vi "HXG2_AlldataToArray.vi"(8 "error in (no error)":errorcluster, 9 "Calculated Values":T1, 10 "Analog In":T2) -> (0 "error out":errorcluster, 2 "Strings Out":string[](array[string])=["Liq In Avg", "Liq In 1", "Liq In 2", "Liq Out Avg", "Liq Out 1", "Liq Out 2", "Fltrd Mdot", "Liq Mdot", "Liq T° f/mtr", "Liq dP 0-25psi", "Liq Pin 0-100psi", "Air In Avg", "Air In 1", "Air In 2", "Air In 3", "Air In 4", "Air Out Avg", "Air Out 1", "Air Out 2", "Air Out 3", "Air Out 4", "Air Out 5", "Air Out 6", "Air Out 7", "Air Out 8", "CFM Nozzle", "CFM HX", "UUT 0-0.1inWC x100", "Chmb 0-5inWC x100", "Chmb 0-2.5inWC x100", "Liq Q (BTU/hr)", "Liq Q (W)", "Air Q (BTU/hr)", "Air Q (W)", "SH (°F)", "SH multiplier", "%Energy Bal", "Liq Re", "AF Ctl Out", "AC Ctl Out", "AH Ctl Out", "LF Ctl Out", "LC Ctl Out", "LH Ctl Out", "Box Btm In (9)", "Box Btm Out (10)", "Box Rt In (11)", "Box Rt Frt (12) ", "Box Top In(13)", "Box Top Out(14)", "Box Lt In (15)", "Box Lt Out (16)"], 3 "Plot":dbl[](array[numeric]))   [LabVIEW 2012]
uses:
  Controls/HXG2_AnalogIn.ctl
  Controls/HXG2_Calculated.ctl
  Modules/PID/HXG2pid.ctl
panel:
  out "element":string
  in  "index":i32=43
  out "Text Array":i32
  out "Number Array":i32
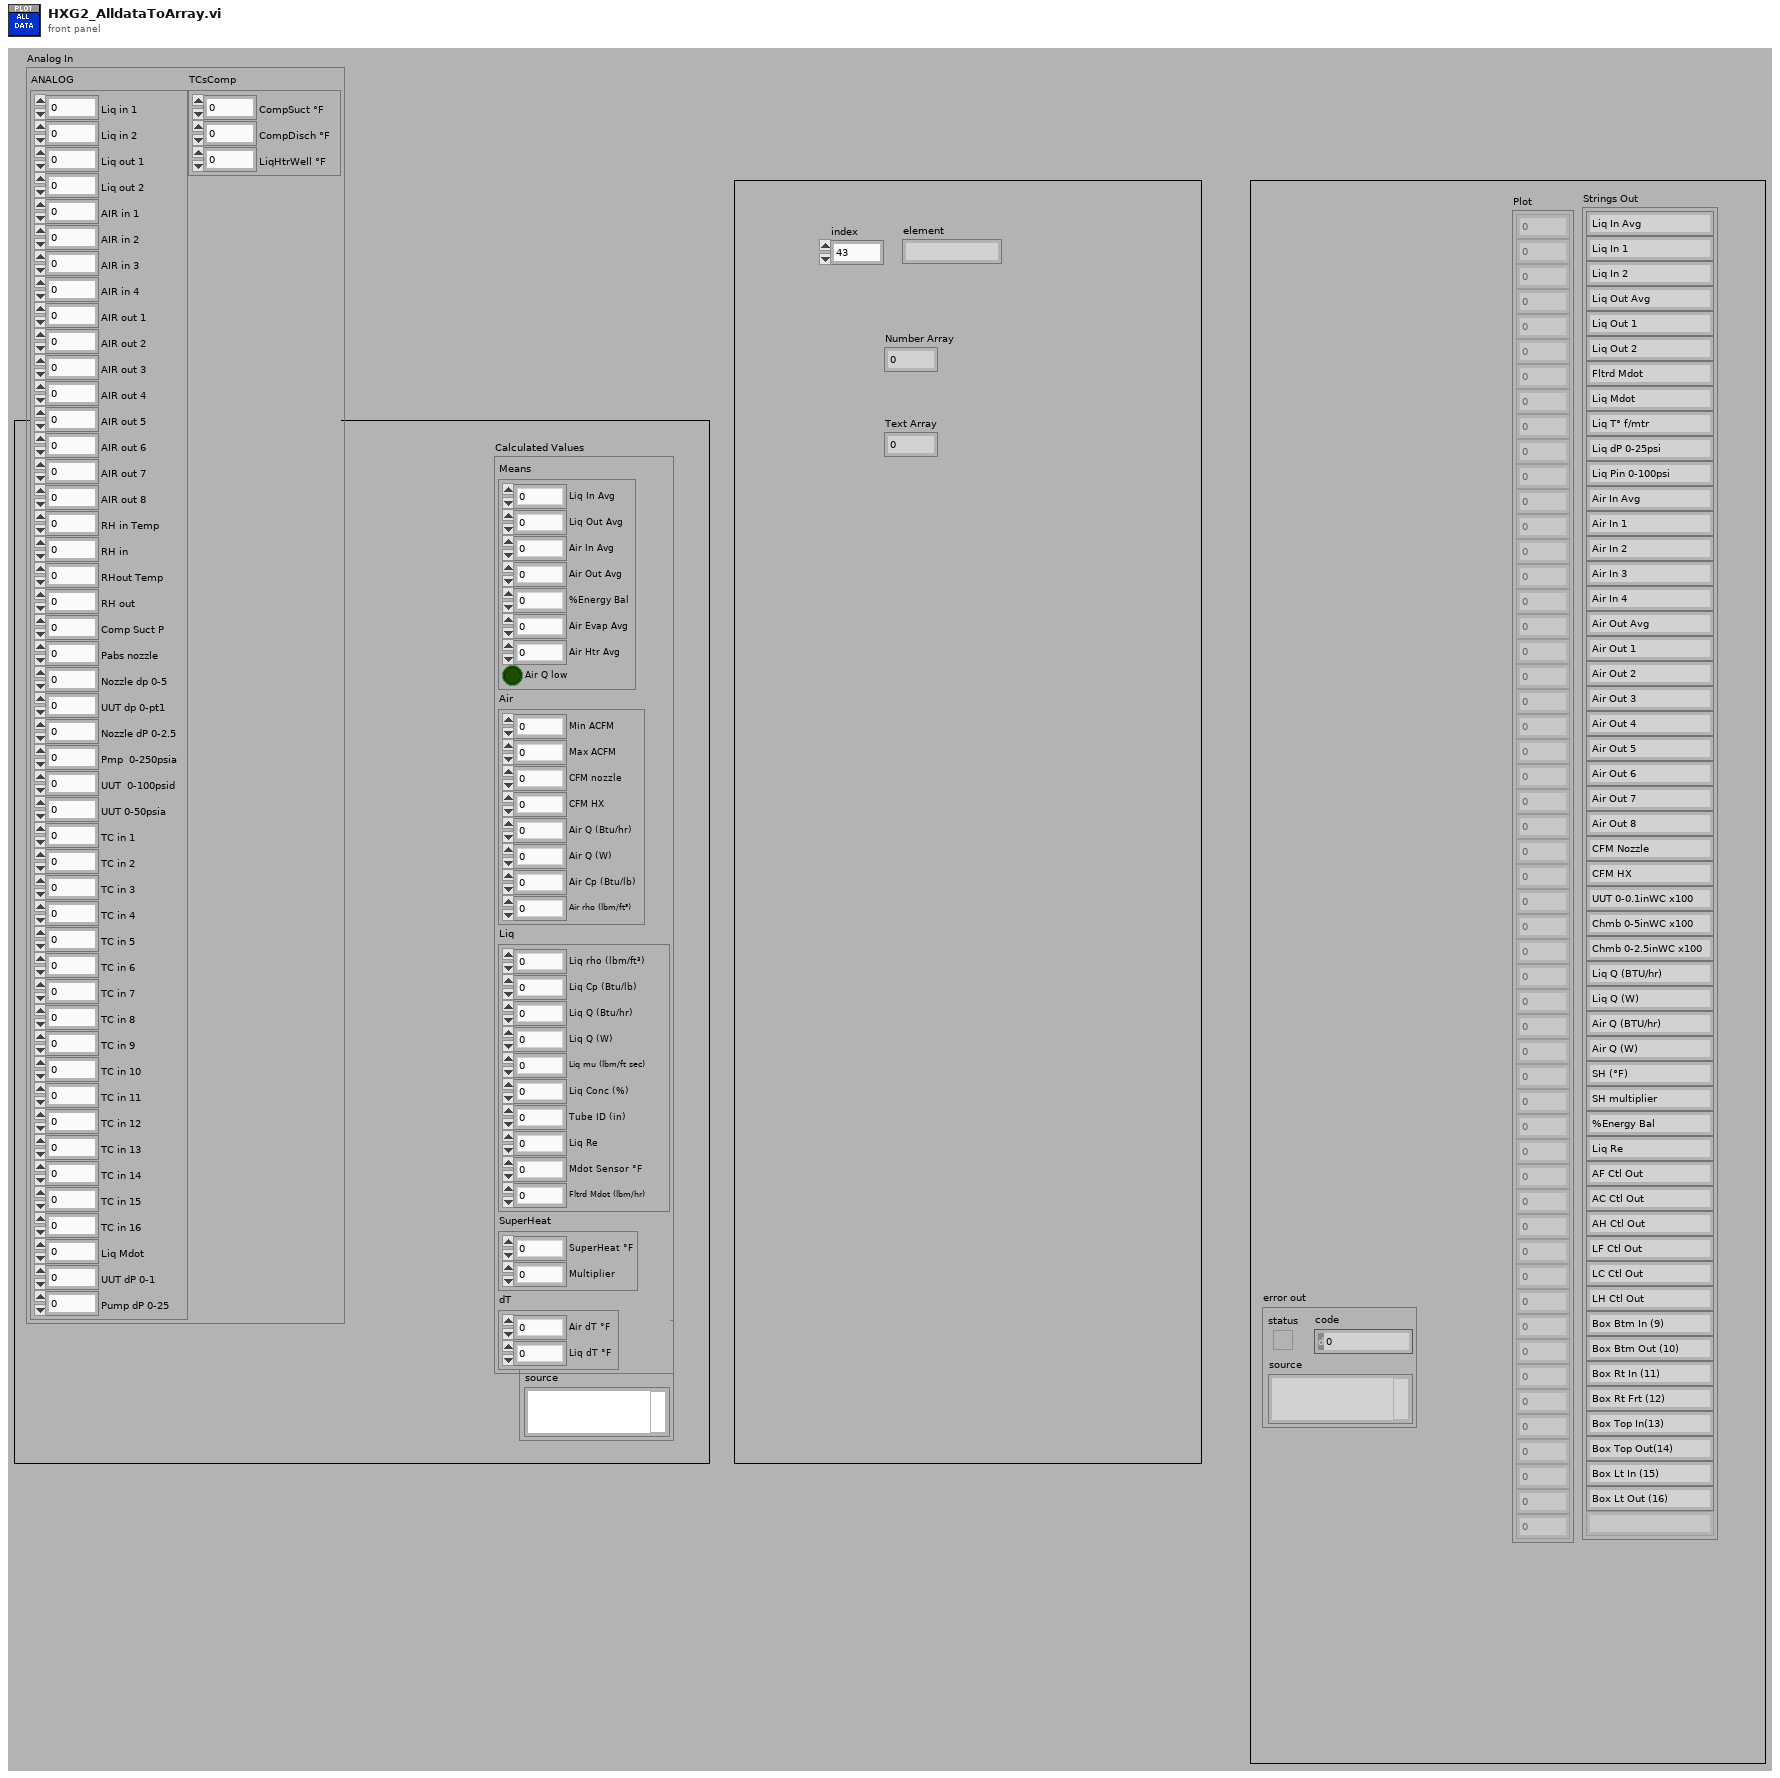
[diagram p1: front panel]
types:
  T1 = typedef "HXG2_Calculated.ctl" = cluster{"Means":cluster{"Liq In Avg":dbl, "Liq Out Avg":dbl, "Air In Avg":dbl, "Air Out Avg":dbl, "%Energy Bal":dbl, "Air Evap Avg":dbl, "Air Htr Avg":dbl, "Air Q low":bool}, "Air":cluster{"Min ACFM":dbl, "Max ACFM":dbl, "CFM nozzle":dbl, "CFM HX":dbl, "Air Q (Btu/hr)":dbl, "Air Q (W)":dbl, "Air Cp (Btu/lb)":dbl, "Air rho (lbm/ft³)":dbl}, "Liq":cluster{"Liq rho (lbm/ft³)":dbl, "Liq Cp (Btu/lb)":dbl, "Liq Q (Btu/hr)":dbl, "Liq Q (W)":dbl, "Liq mu (lbm/ft sec)":dbl, "Liq Conc (%)":dbl, "Tube ID (in)":dbl, "Liq Re":dbl, "Mdot Sensor °F":dbl, "Fltrd Mdot (lbm/hr)":dbl}, "SuperHeat":cluster{"SuperHeat °F":dbl, "Multiplier":dbl}, "dT":cluster{"Air dT °F":dbl, "Liq dT °F":dbl}}
  T2 = typedef "HXG2_AnalogIn.ctl" = cluster{"ANALOG":cluster{"Liq in 1":dbl, "Liq in 2":dbl, "Liq out 1":dbl, "Liq out 2":dbl, "AIR in 1":dbl, "AIR in 2":dbl, "AIR in 3":dbl, "AIR in 4":dbl, "AIR out 1":dbl, "AIR out 2":dbl, "AIR out 3":dbl, "AIR out 4":dbl, "AIR out 5":dbl, "AIR out 6":dbl, "AIR out 7":dbl, "AIR out 8":dbl, "RH in Temp":dbl, "RH in":dbl, "RHout Temp":dbl, "RH out":dbl, "Comp Suct P":dbl, "Pabs nozzle":dbl, "Nozzle dp 0-5":dbl, "UUT dp 0-pt1":dbl, "Nozzle dP 0-2.5":dbl, "Pmp  0-250psia":dbl, "UUT  0-100psid":dbl, "UUT 0-50psia":dbl, "TC in 1":dbl, "TC in 2":dbl, "TC in 3":dbl, "TC in 4":dbl, "TC in 5":dbl, "TC in 6":dbl, "TC in 7":dbl, "TC in 8":dbl, "TC in 9":dbl, "TC in 10":dbl, "TC in 11":dbl, "TC in 12":dbl, "TC in 13":dbl, "TC in 14":dbl, "TC in 15":dbl, "TC in 16":dbl, "Liq Mdot":dbl, "UUT dP 0-1":dbl, "Pump dP 0-25":dbl}, "TCsComp":cluster{"CompSuct °F  ":dbl, "CompDisch °F":dbl, "LiqHtrWell °F":dbl}}
  T3 = typedef "HXG2pid.ctl" = enum16{"Write PID Efforts", "Write PID On-Off", "Pass", "Write PID Refs", "Write PID Gains", "Wrt PID Resets"}
  T4 = typedef "HXG2_PIDctrlsOUT.ctl" = cluster{"Iteration dT (s)":dbl, "af ctrl effort":dbl, "ac ctrl effort":dbl, "ah ctrl effort":dbl, "lf ctrl effort":dbl, "lc ctrl effort":dbl, "lh ctrl effort":dbl}
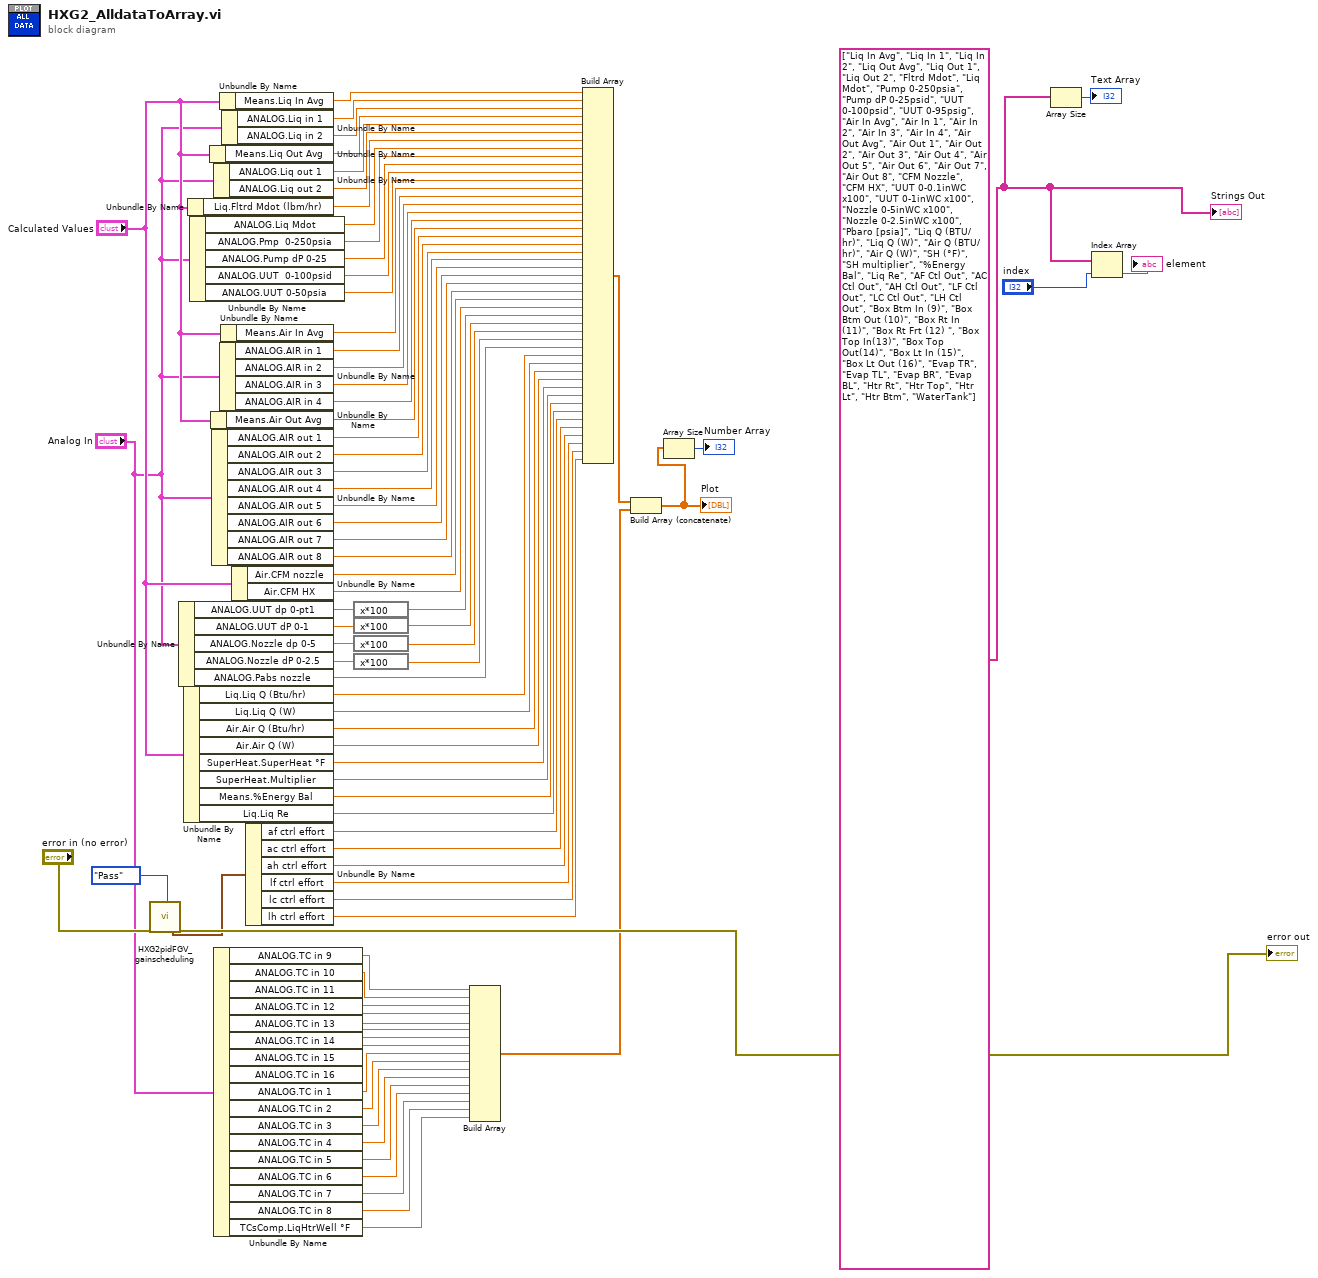
[diagram p0: block diagram]
diagram:
  w6 = string[] ["Liq In Avg", "Liq In 1", "Liq In 2", "Liq Out Avg", "Liq Out 1", "Liq Out 2", "Fltrd Mdot", "Liq Mdot", "Pump 0-250psia", "Pump dP 0-25psid", "UUT 0-100psid", "UUT 0-95psig", "Air In Avg", "Air In 1", "Air In 2", "Air In 3", "Air In 4", "Air Out Avg", "Air Out 1", "Air Out 2", "Air Out 3", "Air Out 4", "Air Out 5", "Air Out 6", "Air Out 7", "Air Out 8", "CFM Nozzle", "CFM HX", "UUT 0-0.1inWC x100", "UUT 0-1inWC x100", "Nozzle 0-5inWC x100", "Nozzle 0-2.5inWC x100", "Pbaro [psia]", "Liq Q (BTU/hr)", "Liq Q (W)", "Air Q (BTU/hr)", "Air Q (W)", "SH (°F)", "SH multiplier", "%Energy Bal", "Liq Re", "AF Ctl Out", "AC Ctl Out", "AH Ctl Out", "LF Ctl Out", "LC Ctl Out", "LH Ctl Out", "Box Btm In (9)", "Box Btm Out (10)", "Box Rt In (11)", "Box Rt Frt (12) ", "Box Top In(13)", "Box Top Out(14)", "Box Lt In (15)", "Box Lt Out (16)", "Evap TR", "Evap TL", "Evap BR", "Evap BL", "Htr Rt", "Htr Top", "Htr Lt", "Htr Btm", "WaterTank"]
  n1 = call "HXG2pidFGV_gainscheduling.vi"("error in (no error)"="error in (no error)", "PIDfgvCtrl"=HXG2pid."Pass") -> ("PID Ctrls Out"=w48:T4, "error out"=→"error out":errorcluster)  [unwired: 9 in, 7 out]
  n2 = Unbundle By Name("Analog In") -> ("ANALOG.UUT dp 0-pt1"=w56:dbl, "ANALOG.UUT dP 0-1"=w8:dbl, "ANALOG.Nozzle dp 0-5"=w37:dbl, "ANALOG.Nozzle dP 0-2.5"=w36:dbl, "ANALOG.Pabs nozzle"=w2:dbl)
  n3 = Unbundle By Name("Calculated Values") -> ("Liq.Liq Q (Btu/hr)"=w3:dbl, "Liq.Liq Q (W)"=w55:dbl, "Air.Air Q (Btu/hr)"=w54:dbl, "Air.Air Q (W)"=w53:dbl, "SuperHeat.SuperHeat °F"=w41:dbl, "SuperHeat.Multiplier"=w38:dbl, "Means.%Energy Bal"=w33:dbl, "Liq.Liq Re"=w32:dbl)
  n4 = Unbundle By Name("Calculated Values") -> ("Liq.Fltrd Mdot (lbm/hr)"=w34:dbl)
  n5 = Unbundle By Name("Analog In") -> ("ANALOG.Liq Mdot"=w62:dbl, "ANALOG.Pmp  0-250psia"=w61:dbl, "ANALOG.Pump dP 0-25"=w9:dbl, "ANALOG.UUT  0-100psid"=w58:dbl, "ANALOG.UUT 0-50psia"=w57:dbl)
  n6 = Unbundle By Name("Calculated Values") -> ("Means.Liq Out Avg"=w79:dbl)
  n7 = Unbundle By Name("Calculated Values") -> ("Means.Air Out Avg"=w71:dbl)
  n8 = Unbundle By Name("Analog In") -> ("ANALOG.AIR out 1"=w70:dbl, "ANALOG.AIR out 2"=w69:dbl, "ANALOG.AIR out 3"=w68:dbl, "ANALOG.AIR out 4"=w67:dbl, "ANALOG.AIR out 5"=w66:dbl, "ANALOG.AIR out 6"=w65:dbl, "ANALOG.AIR out 7"=w64:dbl, "ANALOG.AIR out 8"=w63:dbl)
  n9 = Unbundle By Name("Analog In") -> ("ANALOG.Liq out 1"=w78:dbl, "ANALOG.Liq out 2"=w77:dbl)
  n10 = Unbundle By Name("Analog In") -> ("ANALOG.TC in 9"=w28:dbl, "ANALOG.TC in 10"=w27:dbl, "ANALOG.TC in 11"=w26:dbl, "ANALOG.TC in 12"=w25:dbl, "ANALOG.TC in 13"=w24:dbl, "ANALOG.TC in 14"=w23:dbl, "ANALOG.TC in 15"=w22:dbl, "ANALOG.TC in 16"=w21:dbl, "ANALOG.TC in 1"=w20:dbl, "ANALOG.TC in 2"=w19:dbl, "ANALOG.TC in 3"=w18:dbl, "ANALOG.TC in 4"=w17:dbl, "ANALOG.TC in 5"=w16:dbl, "ANALOG.TC in 6"=w15:dbl, "ANALOG.TC in 7"=w14:dbl, "ANALOG.TC in 8"=w13:dbl, "TCsComp.LiqHtrWell °F"=w1:dbl)
  n11 = Unbundle By Name("Calculated Values") -> ("Means.Liq In Avg"=w82:dbl)
  n12 = Unbundle By Name("Analog In") -> ("ANALOG.AIR in 1"=w75:dbl, "ANALOG.AIR in 2"=w74:dbl, "ANALOG.AIR in 3"=w73:dbl, "ANALOG.AIR in 4"=w72:dbl)
  n13 = Unbundle By Name("Calculated Values") -> ("Means.Air In Avg"=w76:dbl)
  n14 = Unbundle By Name("Analog In") -> ("ANALOG.Liq in 1"=w81:dbl, "ANALOG.Liq in 2"=w80:dbl)
  n15 = Unbundle By Name("Calculated Values") -> ("Air.CFM nozzle"=w60:dbl, "Air.CFM HX"=w59:dbl)
  n16 = Unbundle By Name(w48) -> ("af ctrl effort"=w47:dbl, "ac ctrl effort"=w46:dbl, "ah ctrl effort"=w45:dbl, "lf ctrl effort"=w44:dbl, "lc ctrl effort"=w43:dbl, "lh ctrl effort"=w42:dbl)
  n17 = expression code="x*100"(w56) -> (w40:dbl)
  n18 = expression code="x*100"(w8) -> (w7:dbl)
  n19 = expression code="x*100"(w37) -> (w39:dbl)
  n20 = expression code="x*100"(w36) -> (w35:dbl)
  n21 = Build Array(w28, w27, w26, w25, w24, w23, w22, w21, w20, w19, w18, w17, w16, w15, w14, w13, w1) -> (w11:dbl[])
  n22 = Build Array(w82, w81, w80, w79, w78, w77, w34, w62, w61, w9, w58, w57, w76, w75, w74, w73, w72, w71, w70, w69, w68, w67, w66, w65, w64, w63, w60, w59, w40, w7, w39, w35, w2, w3, w55, w54, w53, w41, w38, w33, w32, w47, w46, w45, w44, w43, w42) -> (w12:dbl[])
  n23 = Build Array (concatenate)(w12, w11) -> (w10:dbl[])
  "Plot" <- w10
  n24 = Array Size(array=w10) -> (size(s)=→"Number Array":i32)
  n25 = Array Size(array=w6) -> (size(s)=→"Text Array":i32)
  n26 = Index Array(array=w6, index="index") -> (element=→"element":string)
  "Strings Out" <- w6
